vi "FPGA_DIOReadLoopTiming.vi"(8 "error in (no error)":errorcluster, 11 "DIODeviceRef In":T1) -> (0 "error out":errorcluster, 2 "LoopTiming":u16, 3 "DIODeviceRef Out":T1)   [LabVIEW 2017]
uses:
  <vilib>/Rock Robotics/SystemInterfaces/DIO/FPGA_DIODevRef.ctl
  <vilib>/Rock Robotics/SystemInterfaces/System/FPGA_SystemFPGA Ref Global.vi
  <vilib>/Utility/error.llb/Error Cluster From Error Code.vi
  <vilib>/rvi/errors/niLvFpgaAdjustHostInterfaceError.vi
  <vilib>/rvi/interface/nirviReadWriteControl/nirviReadWriteControl.xnode
  <vilib>/Rock Robotics/SystemInterfaces/System/FPGA_SystemFRC FPGA Ref.ctl
  NiFpgaLv.dll
  <vilib>/rvi/interface/Simulation/niFpgaSimulationCallBeginRW.vi
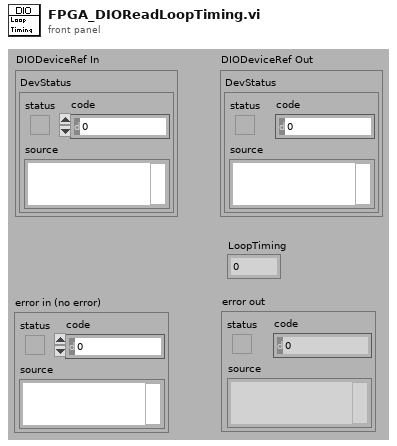
[diagram p1: front panel]
types:
  T1 = typedef "FPGA_DIODevRef.ctl" = cluster{"DevStatus":errorcluster}
  T2 = typedef "FPGA_SystemFRC FPGA Ref.ctl" = refnum<k20>
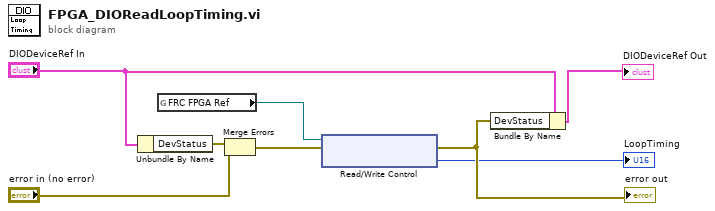
[diagram p0: block diagram]
diagram:
  n1 = Unbundle By Name("DIODeviceRef In") -> ("DevStatus"=w4:errorcluster)
  n2 = global read "FPGA_SystemFPGA Ref Global.vi" "FRC FPGA Ref"() -> (w5:T2)
  n3 = Merge Errors(w4, "error in (no error)") -> (w3:errorcluster)
  n4 = xnode "Read/Write Control"("FPGA VI Reference In"=w5, "error in"=w3) -> ("error out"=w6:errorcluster, "PWM.LoopTiming"=→"LoopTiming":u16)  [unwired: 1 out]
  "error out" <- w6
  n5 = Bundle By Name(cluster="DIODeviceRef In", "DevStatus"=w6) -> (→"DIODeviceRef Out":T1)
